vi "NeedleValveClose.vi"(8 "error in (no error)":errorcluster, 11 "VISA resource name":refnum<visa-resource-name>="ZaberMotor") -> (0 "error out":errorcluster, 3 "VISA resource name out":refnum<visa-resource-name>="ZaberMotor")   [LabVIEW 2018]
uses:
  Request.ctl
  ZaberTSeries.lvlib
panel:
  out "data":dbl
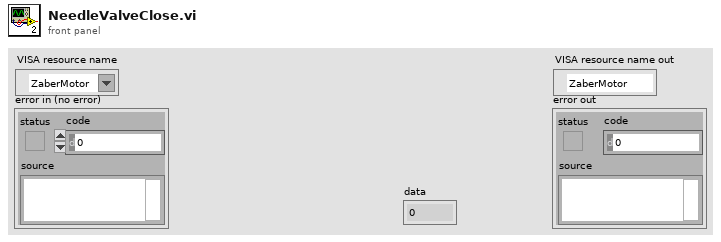
[diagram p1: front panel]
types:
  T1 = typedef "ZaberTSeries.lvlib/Request.ctl" = cluster{"Device Number":u8, "Command":u8, "Data":i32, "Response Count":i32}
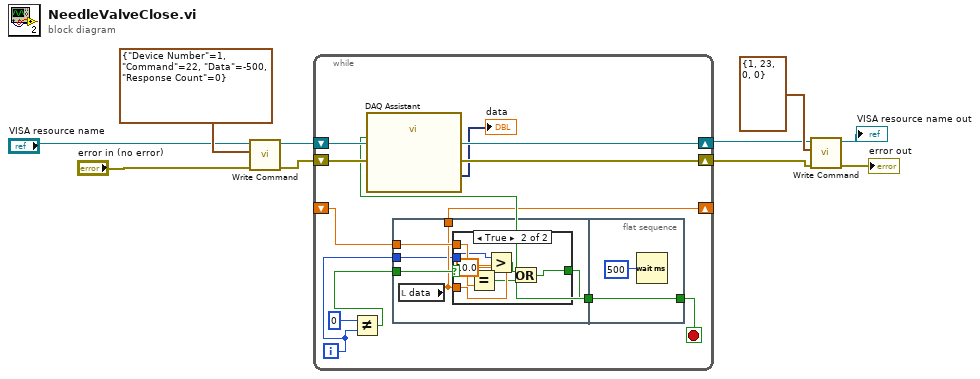
[diagram p0: block diagram]
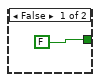
[diagram p2: hidden frame]
diagram:
  n1 = call "Write Command.vi"("error in (no error)"="error in (no error)", "Request"=T1 {"Device Number"=1, "Command"=22, "Data"=-500, "Response Count"=0}, "VISA resource name"="VISA resource name") -> ("error out"=w5:errorcluster, "VISA resource name out"=w6:refnum<visa-resource-name>)  [unwired: 6 in, 1 out]
  n2 = while {
    shift-right: [w20] -> w4
    shift-left: w6 -> [w20]
    shift-right: [w19] -> w3
    shift-left: w5 -> [w19]
    shift-right: [w12] -> _
    shift-left: _ -> [w17]
    i -> [w11]
    stop <- w18 stop-if-true
    n3 = Not Equal?(x=0, y=w11) -> (x != y?=w14:bool)
    n4 = call "DAQ Assistant"("stop (F)"=w18) -> ("data"=→"data":dynamicdata)  [unwired: 15 in, 3 out]
    n5 = flat-sequence {
      tunnel: w17 -> [w24]
      tunnel: w14 -> [w23]
      tunnel: [w25] -> w13
      tunnel: [w22] -> w12
      tunnel: w11 -> [w21]
      tunnel: [w35] -> w18
      tunnel: w13 -> [w35]
      frame #0 {
        n6 = local read "data"() -> (w22:dbl)
        n7 = case shown="True" w23 {
          tunnel: [FALSE w29] -> w25
          tunnel: w24 -> [_ w33]
          tunnel: w22 -> [_ w32]
          tunnel: w21 -> [_ w27]
          frame False {
          }
          frame True {
            n8 = Equal?(x=w32, y=w33) -> (x = y?=w31:bool)
            n9 = Greater?(x=w27, y=10.0) -> (0:w30:bool)
            n10 = Or(x=w30, y=w31) -> (x .or. y?=w29:bool)
          }
        }
      }
      frame #1 {
        n11 = Wait (ms)(milliseconds to wait=u32 500) -> ()  [unwired: 1 out]
      }
    }
  }
  n12 = call "Write Command.vi"("error in (no error)"=w3, "Request"=T1 {"Device Number"=1, "Command"=23, "Data"=0, "Response Count"=0}, "VISA resource name"=w4) -> ("error out"=→"error out":errorcluster, "VISA resource name out"=→"VISA resource name out":refnum<visa-resource-name>)  [unwired: 6 in, 1 out]
